vi "tcp_write_carriers.vi"(8 "Sequence":u32=3 min=1 max=12, 9 "TCP only":bool, 10 "TCP out channels":u32=3 min=1 max=12, 11 "Carrier output":i32[][](array[numeric])) -> (3 "TCP output":bool)   [LabVIEW 2014]
uses:
  ilemt_globals.vi
panel:
  out "Bad":bool
  out "error out":errorcluster
  out "bytes written":i32
  out "Out buffer":i32[](array[numeric])
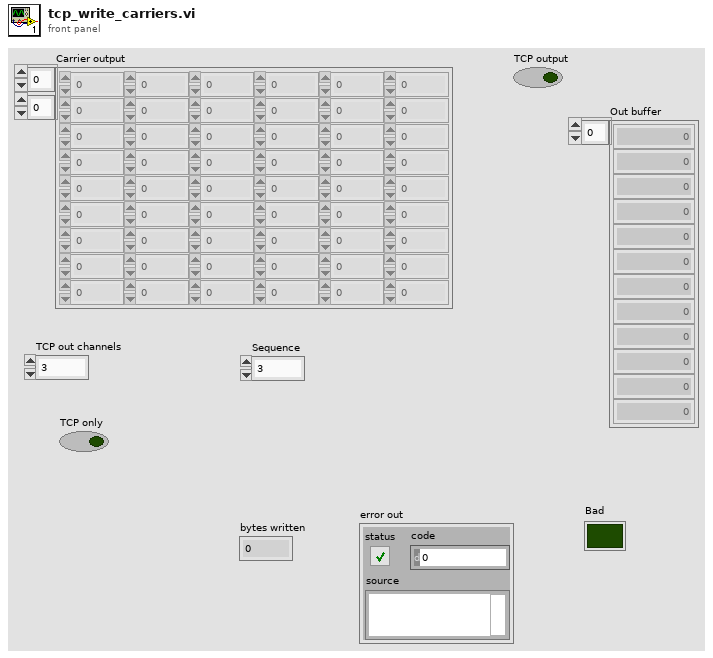
[diagram p1: front panel]
types:
  T1 = enum16{"big-endian, network order", "native, host order", "little-endian"}
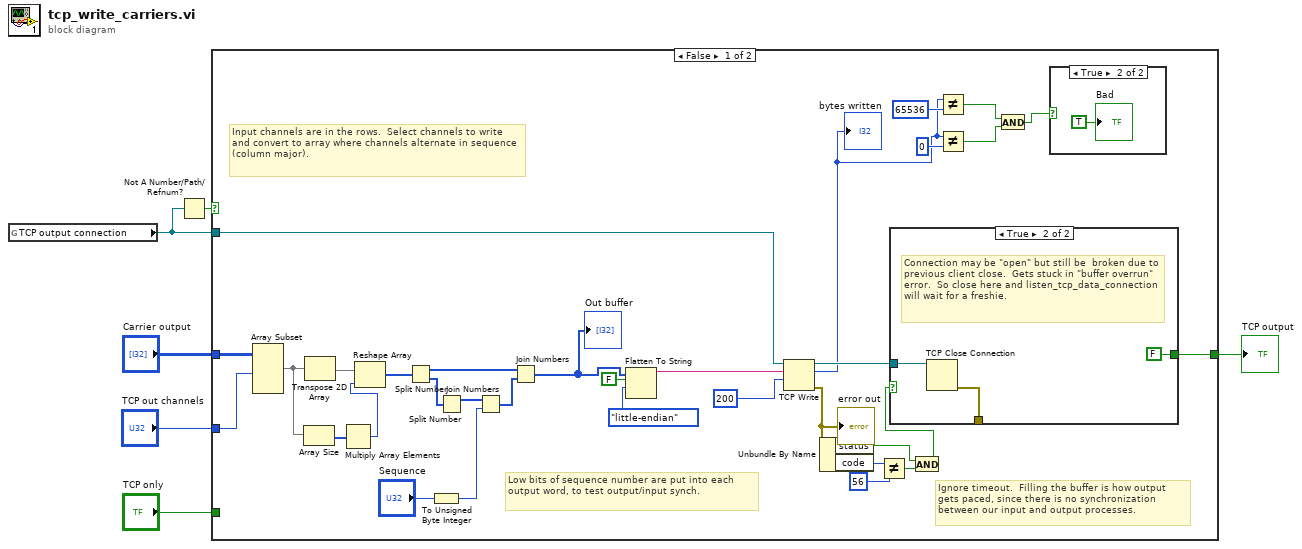
[diagram p0: block diagram]
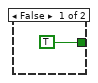
[diagram p3: hidden frame]
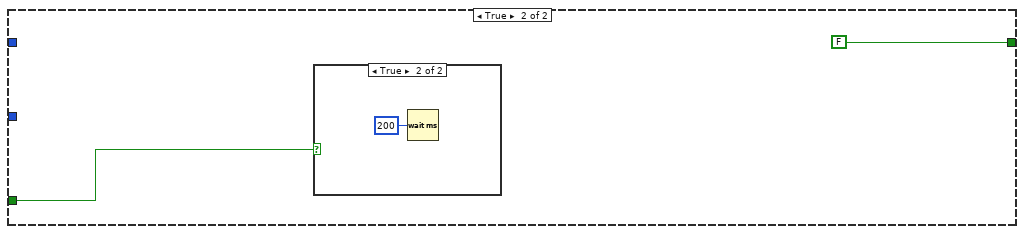
[diagram p4: hidden frame]
diagram:
  n1 = global read "ilemt_globals.vi" "TCP output connection"() -> (w4:refnum<k5>)
  n2 = Not A Number/Path/Refnum?(number/path/refnum=w4) -> (NaN/Path/Refnum?=w5:bool)
  n3 = case shown="False" w5 {
    tunnel: "Carrier output" -> [w26 _]
    tunnel: w4 -> [w38 _]
    tunnel: [w37 FALSE ("TCP output")] -> w3
    tunnel: "TCP only" -> [_ w45]
    tunnel: "TCP out channels" -> [w25 _]
    frame False {
      # "Low bits of sequence number are put into each output word, to test output/input synch."
      # "Input channels are in the rows.  Select channels to write and convert to array where channels alternate in sequence (column major)."
      # "Ignore timeout.  Filling the buffer is how output gets paced, since there is no synchronization between our input and output processes."
      n4 = Array Subset(array=w26, length (row)=w25) -> (w23:i32[][])  [unwired: 3 in]
      n5 = Array Size(array=w23) -> (size(s)=w22:i32[])
      n6 = Transpose 2D Array(2D array=w23) -> (transposed array=w24:i32[][])
      n7 = Multiply Array Elements(1:w22) -> (0:w21:i32)
      n8 = Reshape Array(w24, w21) -> (w14:i32[])
      n9 = Split Number(x=w14) -> (hi(x)=w11:u16[], lo(x)=w13:u16[])
      n10 = To Unsigned Byte Integer(number="Sequence") -> (unsigned 8bit integer=w8:u8)
      n11 = Split Number(x=w13) -> (hi(x)=w9:u8[])  [unwired: 1 out]
      n12 = Join Numbers(hi=w9, lo=w8) -> ((hi.lo)=w10:u16[])
      n13 = Join Numbers(hi=w11, lo=w10) -> ((hi.lo)=w7:u32[])
      "Out buffer" <- w7
      n14 = Flatten To String(anything=w7, prepend array or string size? (T)=FALSE, byte order (0:big-endian, network order)=T1."little-endian") -> (data string=w27:string)  [unwired: 1 in, 2 out]
      n15 = TCP Write(connection ID=w38, data in=w27, 9:200 ("timeout ms (25000)")) -> (connection ID out=w36:refnum<k5>, bytes written=w18:i32, error out=w33:errorcluster)  [unwired: 1 in]
      "bytes written" <- w18
      "error out" <- w33
      n16 = Unbundle By Name(w33) -> ("status"=w29:bool, "code"=w32:i32)
      n17 = Not Equal?(x=w32, y=56) -> (x != y?=w30:bool)
      n18 = And(x=w29, y=w30) -> (x .and. y?=w28:bool)
      n19 = case shown="True" w28 {
        tunnel: [TRUE ("TCP output") FALSE ("TCP output")] -> w37
        tunnel: w36 -> [_ w43]
        tunnel: [_ w42] -> _
        frame False {
        }
        frame True {
          # "Connection may be \"open\" but still be  broken due to previous client close.  Gets stuck in \"buffer overrun\" error.  So close here and listen_tcp_data_connection will wait for a freshie."
          n20 = TCP Close Connection(connection ID=w43) -> (error out=w42:errorcluster)  [unwired: 1 in, 2 out]
        }
      }
      n21 = Not Equal?(x=w18, y=65536) -> (x != y?=w16:bool)
      n22 = Not Equal?(x=w18, y=0) -> (x != y?=w17:bool)
      n23 = And(x=w16, y=w17) -> (x .and. y?=w15:bool)
      n24 = case shown="True" w15 {
        frame False {
        }
        frame True {
          "Bad" <- TRUE ("Bad")
        }
      }
    }
    frame True {
      n25 = case shown="True" w45 {
        frame False {
        }
        frame True {
          n26 = Wait (ms)(milliseconds to wait=u32 200) -> ()  [unwired: 1 out]
        }
      }
    }
  }
  "TCP output" <- w3
